vi "scd41-csv-to-data.vi"(10 "sensor-name":string, 11 "sensor-csv-input":string) -> (0 "SCD41: Humidity (%)":dbl format="%.2f", 1 "SCD41: Temp (degC)":dbl format="%.2f", 2 "SCD41: CO2 (ppm)":dbl format="%.2f", 3 "SCD typedef":T1 {"Humidity (%)" format="%.2f"; "Temp (degC)" format="%.2f"; "CO2 (ppm)" format="%.2f"})   [LabVIEW 2021]
uses:
  SCD41.ctl
  <vilib>/regexp/Match Regular Expression.xnode
panel:
  out "CD1: Humidity":string
  out "SCD41: Temp":string
  out "SCD41: CO2":string
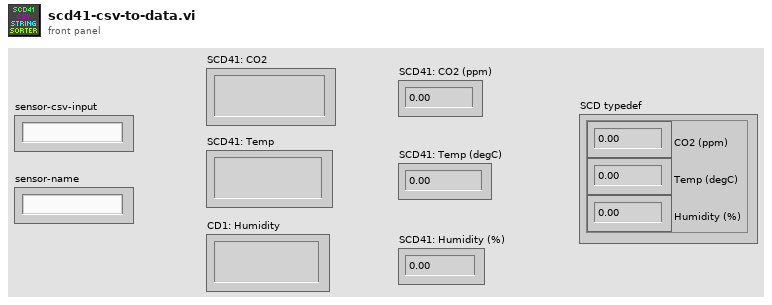
[diagram p1: front panel]
types:
  T1 = typedef "SCD41.ctl" = cluster{"CO2 (ppm)":dbl, "Temp (degC)":dbl, "Humidity (%)":dbl}
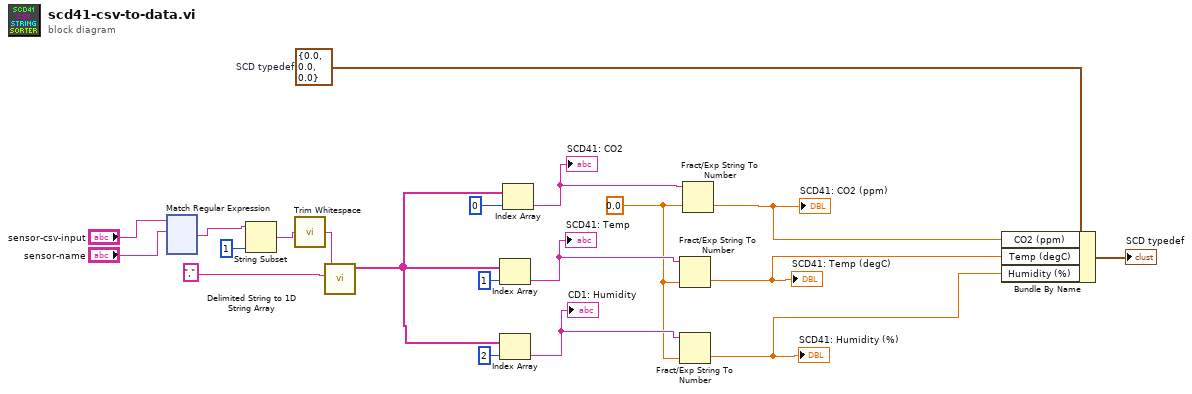
[diagram p0: block diagram]
diagram:
  w9 = T1 {"CO2 (ppm)"=0.0, "Temp (degC)"=0.0, "Humidity (%)"=0.0}  # SCD typedef
  w5 = 0.0
  n1 = xnode "Match Regular Expression"("input string"="sensor-csv-input", "regular expression"="sensor-name") -> ("after match"=w3:string)  [unwired: 4 in, 4 out]
  n2 = String Subset(string=w3, offset (0)=1) -> (substring=w2:string)  [unwired: 1 in]
  n3 = call <vilib>:"Trim Whitespace.vi"("string"=w2) -> ("trimmed string"=w20:string)  [unwired: 1 in]
  n4 = call <vilib>:"Delimited String to 1D String Array.vi"("delimiter"=",", "delimited string"=w20) -> ("string array"=w4:string[])  [unwired: 9 in]
  n5 = Index Array(array=w4, index=1) -> (element=w15:string)
  "SCD41: Temp" <- w15
  n6 = Index Array(array=w4, index=2) -> (element=w16:string)
  "CD1: Humidity" <- w16
  n7 = Index Array "Index Array"(array=w4, index=0) -> (element=w14:string)
  "SCD41: CO2" <- w14
  n8 = Fract/Exp String To Number(string=w15, default (0 dbl)=w5) -> (number=w12:dbl)  [unwired: 2 in, 1 out]
  "SCD41: Temp (degC)" <- w12
  n9 = Fract/Exp String To Number(string=w16, default (0 dbl)=w5) -> (number=w13:dbl)  [unwired: 2 in, 1 out]
  "SCD41: Humidity (%)" <- w13
  n10 = Fract/Exp String To Number(string=w14, default (0 dbl)=w5) -> (number=w11:dbl)  [unwired: 2 in, 1 out]
  "SCD41: CO2 (ppm)" <- w11
  n11 = Bundle By Name(cluster=w9, "CO2 (ppm)"=w11, "Temp (degC)"=w12, "Humidity (%)"=w13) -> (→"SCD typedef":T1)
